vi "TestExec.Merge INI Files.vi"(8 "error in":errorcluster, 10 "Dest File":path, 11 "Source File":path) -> (0 "error out":errorcluster, 3 "Files":path[](array[path]))   [LabVIEW 2018]
uses:
  <vilib>/Utility/config.llb/Read Key (String).vi
  <vilib>/Utility/config.llb/Write Key (String).vi
  <vilib>/Utility/config.llb/NI_LVConfig.lvlib
panel:
  in  "Additional Config Section Names":string[](array[string])=["AdditionalConfig", "Station"]
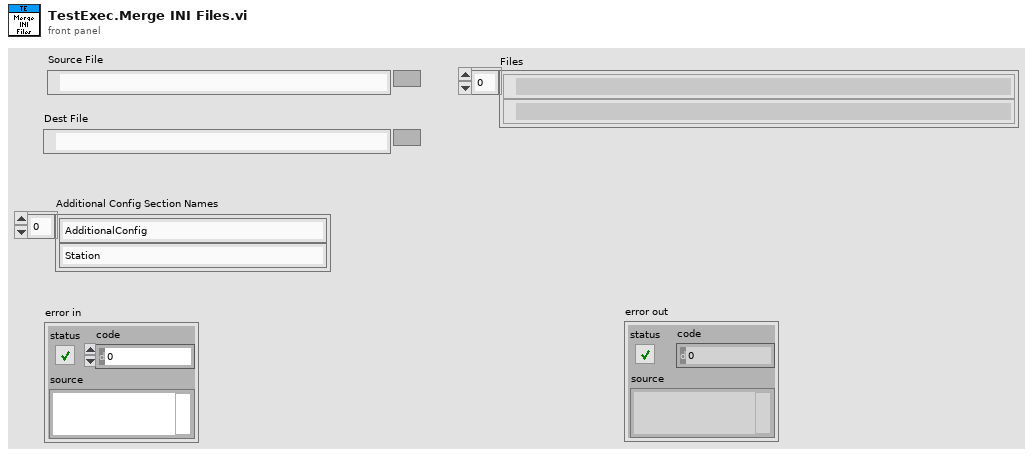
[diagram p1: front panel]
types:
  T1 = typedef "NI_LVConfig.lvlib/Config Data RefNum.ctl" = refnum<k1>
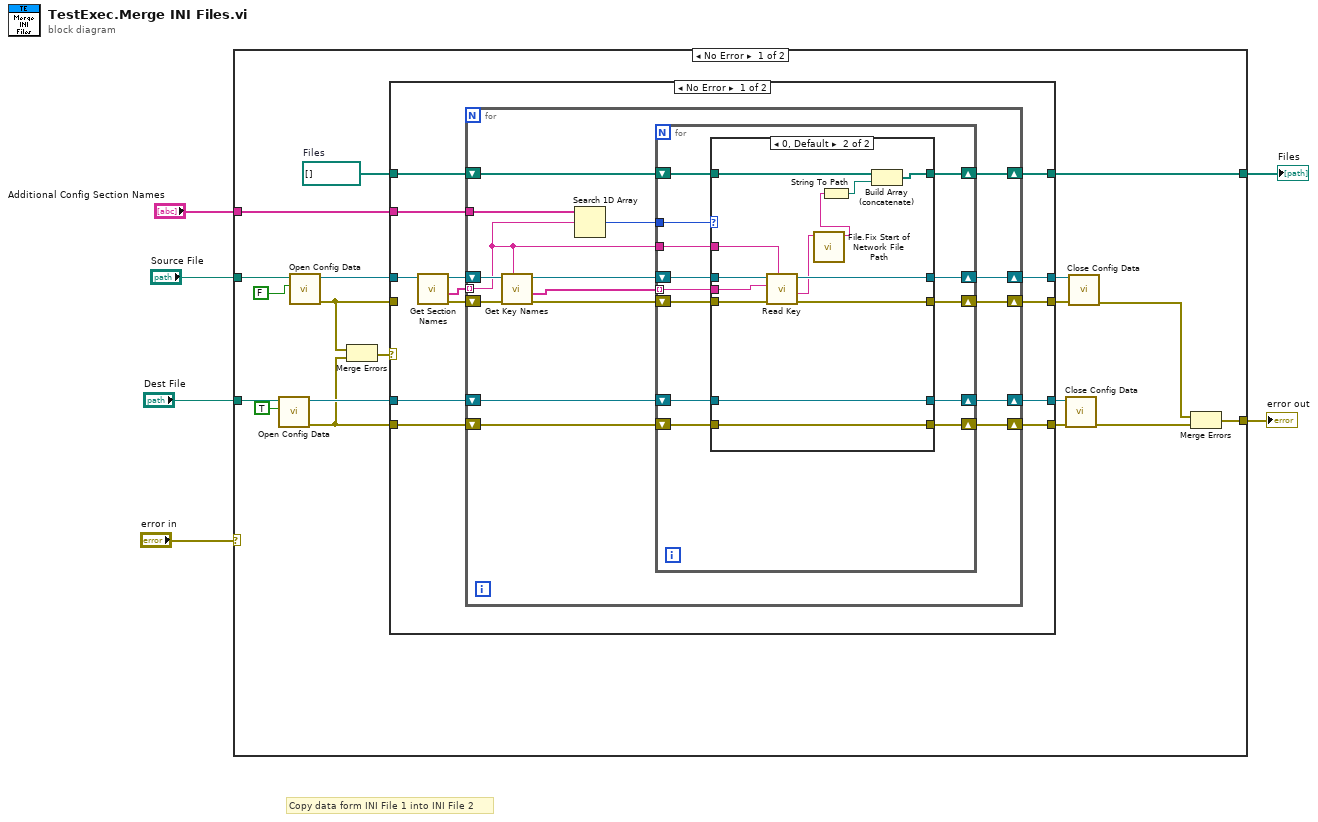
[diagram p0: block diagram]
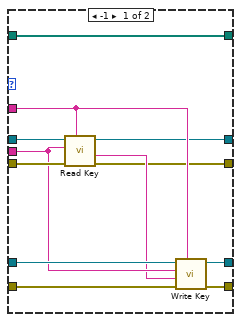
[diagram p2: hidden frame]
diagram:
  # "Copy data form INI File 1 into INI File 2"
  n1 = case shown="No Error" "error in" {
    selector: "error in" -> [_ w98]
    tunnel: [w13 w98] -> w5
    tunnel: "Source File" -> [w25 _]
    tunnel: "Dest File" -> [w22 _]
    tunnel: "Additional Config Section Names" -> [w11 _]
    tunnel: [w10 _] -> w1
    frame No Error {
      w12 = path[] []  # Files
      n2 = call <vilib>:"Open Config Data.vi"("create file if necessary (T)"=TRUE, "configuration file path"=w22) -> ("error out"=w20:errorcluster, "refnum"=w21:T1)  [unwired: 7 in, 1 out]
      n3 = call <vilib>:"Open Config Data.vi"("create file if necessary (T)"=FALSE, "configuration file path"=w25) -> ("error out"=w8:errorcluster, "refnum"=w23:T1)  [unwired: 7 in, 1 out]
      n4 = Merge Errors(w8, w20) -> (w9:errorcluster)
      n5 = case shown="No Error" w9 {
        tunnel: w23 -> [w38 w97]
        tunnel: w21 -> [w34 w96]
        tunnel: w20 -> [w33 w95]
        tunnel: [w32 w95] -> w17
        tunnel: [w31 w94] -> w18
        tunnel: [w30 w97] -> w19
        tunnel: [w29 w96] -> w16
        tunnel: w12 -> [w28 w93]
        tunnel: w11 -> [w27 _]
        tunnel: [w26 w93] -> w10
        tunnel: w8 -> [_ w94]
        frame No Error {
          n6 = call <vilib>:"Get Section Names.vi"("refnum"=w38) -> ("error out"=w35:errorcluster, "section names"=w37:string[], "refnum out"=w36:T1)  [unwired: 8 in]
          n7 = for {
            tunnel: w37 -> [w39] mode=indexing
            shift-right: [w47] -> w31
            shift-left: w35 -> [w54]
            shift-right: [w46] -> w32
            shift-left: w33 -> [w48]
            shift-right: [w45] -> w30
            shift-left: w36 -> [w53]
            shift-right: [w44] -> w29
            shift-left: w34 -> [w49]
            shift-right: [w41] -> w26
            shift-left: w28 -> [w43]
            tunnel: w27 -> [w42]
            n8 = call <vilib>:"Get Key Names.vi"("section"=w39, "error in (no error)"=w54, "refnum"=w53) -> ("error out"=w51:errorcluster, "key names"=w50:string[], "refnum out"=w52:T1)  [unwired: 5 in, 1 out]
            n9 = Search 1D Array(1D array=w42, element=w39) -> (index of element=w40:i32)  [unwired: 1 in]
            n10 = for {
              tunnel: w50 -> [w57] mode=indexing
              tunnel: w39 -> [w64]
              shift-right: [w63] -> w46
              shift-left: w48 -> [w62]
              shift-right: [w61] -> w47
              shift-left: w51 -> [w66]
              shift-right: [w60] -> w45
              shift-left: w52 -> [w67]
              shift-right: [w59] -> w44
              shift-left: w49 -> [w65]
              shift-right: [w56] -> w41
              shift-left: w43 -> [w58]
              tunnel: w40 -> [w55]
              n11 = case shown="0, Default" w55 {
                tunnel: w67 -> [w79 w92]
                tunnel: w66 -> [w78 w91]
                tunnel: w65 -> [w77 w86]
                tunnel: w64 -> [w76 w90]
                tunnel: w57 -> [w75 w89]
                tunnel: [w73 w85] -> w63
                tunnel: w62 -> [w72 w85]
                tunnel: [w71 w88] -> w61
                tunnel: [w70 w87] -> w60
                tunnel: [w69 w86] -> w59
                tunnel: w58 -> [w68 w84]
                tunnel: [w68 w83] -> w56
                frame -1 {
                  n12 = call-poly <vilib>:"Read Key.vi"("section"=w76, "error in (no error)"=w78, "key"=w75, "refnum"=w79) -> ("error out"=w71:errorcluster, "value"=w74:string, "refnum out"=w70:T1)  [unwired: 4 in, 1 out]
                  n13 = call-poly <vilib>:"Write Key.vi"("section"=w76, "error in (no error)"=w72, "value"=w74, "key"=w75, "refnum"=w77) -> ("error out"=w73:errorcluster, "refnum out"=w69:T1)  [unwired: 4 in, 1 out]
                }
                frame 0, Default {
                  n14 = call-poly <vilib>:"Read Key.vi"("section"=w90, "error in (no error)"=w91, "key"=w89, "refnum"=w92) -> ("error out"=w88:errorcluster, "value"=w81:string, "refnum out"=w87:T1)  [unwired: 4 in, 1 out]
                  n15 = call "File.Fix Start of Network File Path.vi"("String Path"=w81) -> ("String Path Out"=w80:string)  [unwired: 10 in]
                  n16 = String To Path(string=w80) -> (path=w82:path)
                  n17 = Build Array (concatenate)(w84, w82) -> (w83:path[])
                }
              }
            }
          }
        }
        frame Error {
        }
      }
      n18 = call <vilib>:"Close Config Data.vi"("error in (no error)"=w17, "refnum"=w16) -> ("error out"=w14:errorcluster)  [unwired: 8 in, 1 out]
      n19 = call <vilib>:"Close Config Data.vi"("error in (no error)"=w18, "refnum"=w19) -> ("error out"=w15:errorcluster)  [unwired: 8 in, 1 out]
      n20 = Merge Errors(w15, w14) -> (w13:errorcluster)
    }
    frame Error {
    }
  }
  "error out" <- w5
  "Files" <- w1
